vi "DG535.GetActDelay.vi"(0 "i ref in":refnum<vi>, 5 "error in (no error)":errorcluster) -> (14 "i ref out":refnum<vi>, 16 "ActDelay":dbl format="%.2f", 19 "error out":errorcluster)   [LabVIEW 2014, in "DG535.lvlib"]
uses:
  DG535.lvlib
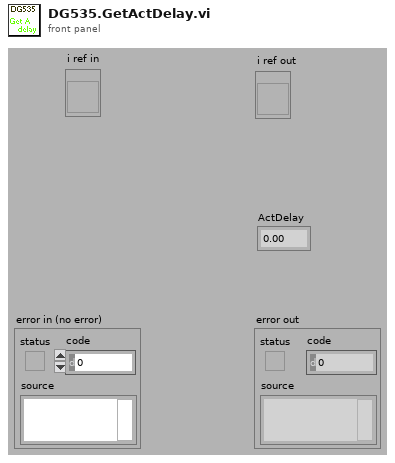
[diagram p1: front panel]
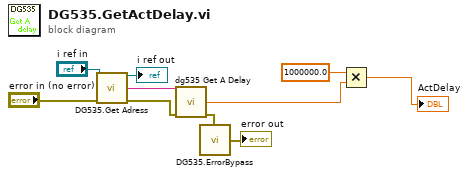
[diagram p0: block diagram]
diagram:
  n1 = call "DG535.Get Adress.vi"("i ref in"="i ref in", "error in (no error)"="error in (no error)") -> ("i ref out"=→"i ref out":refnum<vi>, "address"=w7:string, "error out"=w6:errorcluster)  [unwired: 10 in, 1 out]
  n2 = call "dg535 Get A Delay.vi"("address string"=w7, "error in"=w6) -> ("A"=w2:dbl, "error out"=w5:errorcluster)  [unwired: 11 in, 1 out]
  n3 = call "DG535.ErrorBypass.vi"("error in (no error)"=w5) -> ("error out"=→"error out":errorcluster)  [unwired: 14 in]
  n4 = Multiply(x=1000000.0, y=w2) -> (x*y=→"ActDelay":dbl)
